vi "TemperatureOnly.vi"() -> ()   [LabVIEW 2014]
uses:
  <vilib>/Utility/error.llb/DialogType.ctl
  <instrlib>/Fluke 884X Series/Public/Data/Read (Multiple Points).vi
  <vilib>/Utility/file.llb/Write To Spreadsheet File (DBL).vi
  <instrlib>/Fluke 884X Series/Fluke 884X Series.lvlib
panel:
  in  "stop":bool
  in  "Write":bool
  in  "Serial Configuration":T1={"Baud Rate"=9600, "Parity"=0, "Data Bits"=8, "Stop Bits"=10, "Flow Control"=0} {"Flow Control" items=["None", "XON/XOFF", "RTS/CTS", "XON/XOFF & RTS/CTS", "DTR/DSR", "XON/XOFF & DTR/DSR"]; "Stop Bits" items=["1.0"=10, "1.5"=15, "2.0"=20]; "Data Bits" items=["7"=7, "8"=8]; "Parity" items=["None", "Odd", "Even", "Mark", "Space"]; "Baud Rate" items=["300"=300, "600"=600, "1200"=1200, "2400"=2400, "4800"=4800, "9600"=9600, "19200"=19200]}
  in  "VISA resource name":refnum<visa-resource-name>
  in  "mkv per degree(thermocouple type)":dbl
  out "T,C":dbl
  out "T,K":dbl
  in  "Tkomn, C":dbl
  in  "Timeout":i32=10000
  in  "Sample Count (10)":i32=10
  in  "Manual Range (1.0)":dbl=1.0
  in  "Auto Range (T:Enable)":bool=TRUE
  in  "Function (0: DC Voltage)":u16(ring) items=["DC Voltage", "AC Voltage", "2 - Wire Resistance", "4 - Wire Resistance", "DC Current", "AC Current", "Frequency", "Period", "Continuity", "Diode Checking", "Temperature", "Capacitance"]
  in  "Manual Resolution (5.5 Digits)":dbl(ring)=5.5 items=["4.5"=4.5, "5.5"=5.5, "6.5"=6.5]
  out "Temperature":dbl
  out "Temperature from Fluke884X":dbl[](graph)
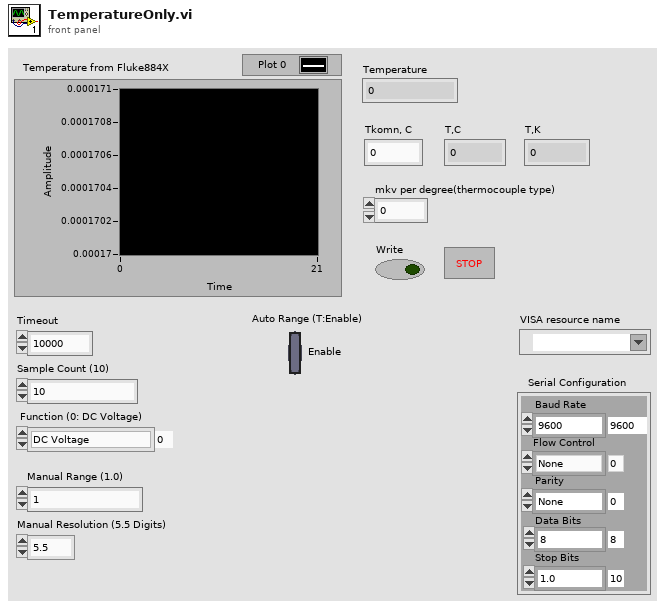
[diagram p1: front panel]
types:
  T1 = cluster{"Baud Rate":u32, "Parity":u16, "Data Bits":u16, "Stop Bits":u16, "Flow Control":u16}
  T2 = typedef "DialogType.ctl" = u16
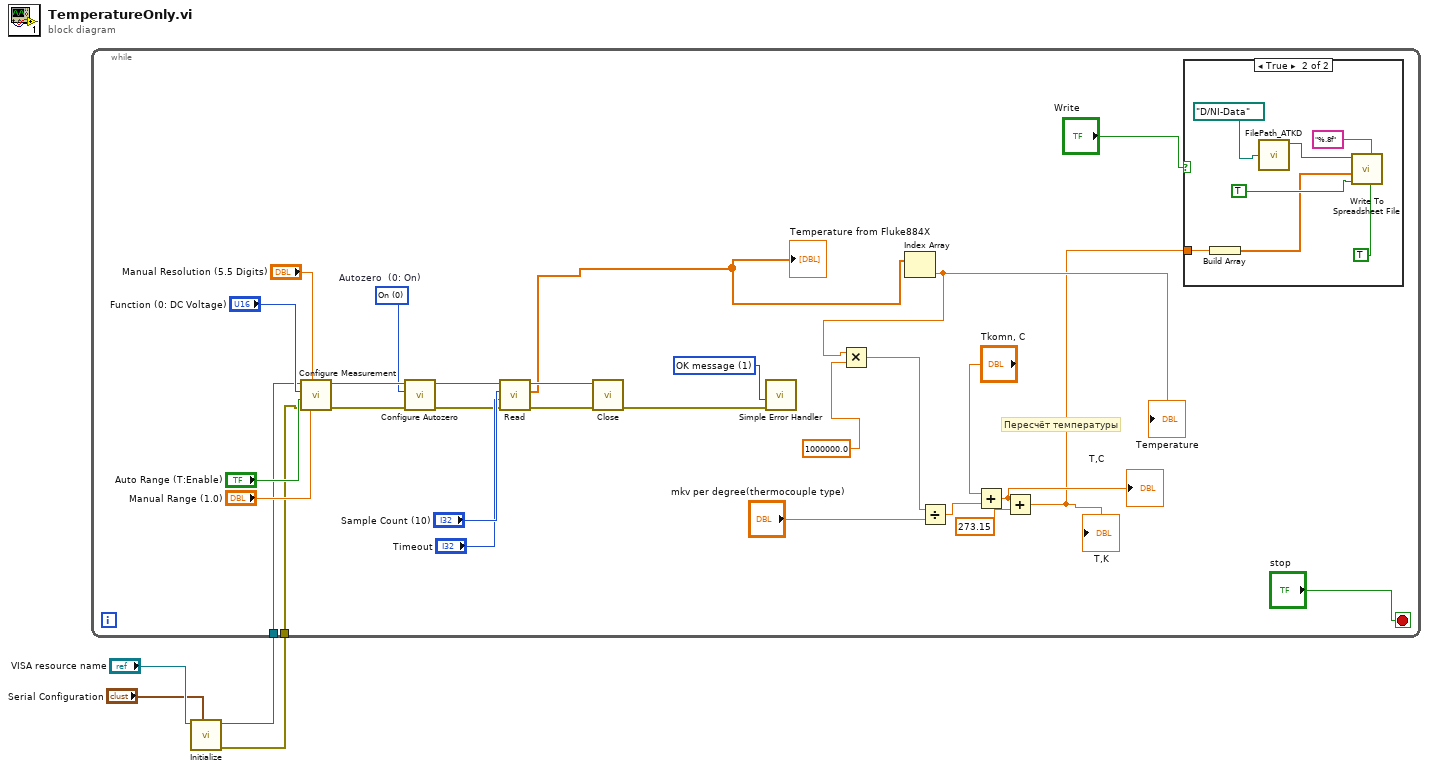
[diagram p0: block diagram]
diagram:
  n1 = call <instrlib>:"Initialize.vi"("Serial Configuration"="Serial Configuration", "VISA resource name"="VISA resource name") -> ("error out"=w1:errorcluster, "VISA resource name out"=w2:refnum<visa-resource-name>)  [unwired: 8 in]
  n2 = while {
    tunnel: w2 -> [w9]
    tunnel: w1 -> [w8]
    stop <- "stop" stop-if-true
    w19 = u16 0 items=["On", "Off", "Once"]  # Autozero  (0: On)
    w33 = T2 1 items=["no dialog", "OK message", "continue or stop message", "OK message + warnings", "continue/stop + warnings"] ("type of dialog (OK msg:1)")
    # "Пересчёт температуры"
    n3 = call <instrlib>:"Configure Measurement.vi"("Manual Range (1.0)"="Manual Range (1.0)", "Manual Resolution (5.5 Digits)"="Manual Resolution (5.5 Digits)", "error in (no error)"=w8, "Auto Range (T:Enable)"="Auto Range (T:Enable)", "Function (0: DC Voltage)"="Function (0: DC Voltage)", "VISA resource name"=w9) -> ("error out"=w23:errorcluster, "VISA resource name out"=w22:refnum<visa-resource-name>)  [unwired: 4 in]
    n4 = call <instrlib>:"Configure Autozero.vi"("error in (no error)"=w23, "Autozero  (0: On)"=w19, "VISA resource name"=w22) -> ("error out"=w20:errorcluster, "VISA resource name out"=w21:refnum<visa-resource-name>)  [unwired: 7 in]
    n5 = call-poly <instrlib>:"Read.vi"("error in (no error)"=w20, "Timeout (10000 ms)"="Timeout", "Sample Count (1)"="Sample Count (10)", "VISA resource name"=w21) -> ("error out"=w30:errorcluster, "Measurements"=w14:dbl[], "VISA resource name out"=w31:refnum<visa-resource-name>)  [unwired: 5 in]
    "Temperature from Fluke884X" <- w14
    n6 = call <instrlib>:"Close.vi"("error in (no error)"=w30, "VISA resource name"=w31) -> ("error out"=w32:errorcluster)  [unwired: 9 in]
    n7 = call <vilib>:"Simple Error Handler.vi"("type of dialog (OK msg:1)"=w33, "error in (no error)"=w32) -> ()  [unwired: 3 in, 5 out]
    n8 = Index Array(array=w14) -> (element=w12:dbl)  [unwired: 1 in]
    "Temperature" <- w12
    n9 = Multiply(x=w12, y=1000000.0) -> (x*y=w10:dbl)
    n10 = Divide(x=w10, y="mkv per degree(thermocouple type)") -> (x/y=w17:dbl)
    n11 = Add(x="Tkomn, C", y=w17) -> (x+y=w15:dbl)
    "T,C" <- w15
    n12 = Add(x=w15, y=273.15) -> (x+y=w6:dbl)
    "T,K" <- w6
    n13 = case shown="True" "Write" {
      tunnel: w6 -> [_ w35]
      frame False {
      }
      frame True {
        n14 = Build Array(w35) -> (w34:dbl[])
        n15 = call "FilePath_ATKD.vi"("base folder path"=path "D:/NI-Data") -> ("ATKD"=w38:path)  [unwired: 3 out]
        n16 = call-poly <vilib>:"Write To Spreadsheet File.vi"("transpose? (no:F)"=TRUE ("append to file? (new file:F)"), "format (%.3f)"="%.8f", "append to file? (new file:F)"=TRUE, "1D data"=w34, "file path (dialog if empty)"=w38) -> ()  [unwired: 1 in, 3 out]
      }
    }
  }
